vi "Main.vi"(8 "error in (no error)":errorcluster, 11 "Transceiver Thread in":refnum<class "Transceiver Thread.lvclass">) -> (0 "error out":errorcluster, 3 "Transceiver Thread out":refnum<class "Transceiver Thread.lvclass">)   [LabVIEW 2017, in "DSF Core.lvlib" / "Transceiver Thread.lvclass"]
uses:
  Transceiver Thread.lvclass
  C:/Git/DSF/Core/Classes/Thread/Plugin/Plugin Thread.lvclass
  C:/Git/DSF/Core/Classes/Thread/Thread.lvclass
  Thread.lvclass
  Plugin Thread.lvclass
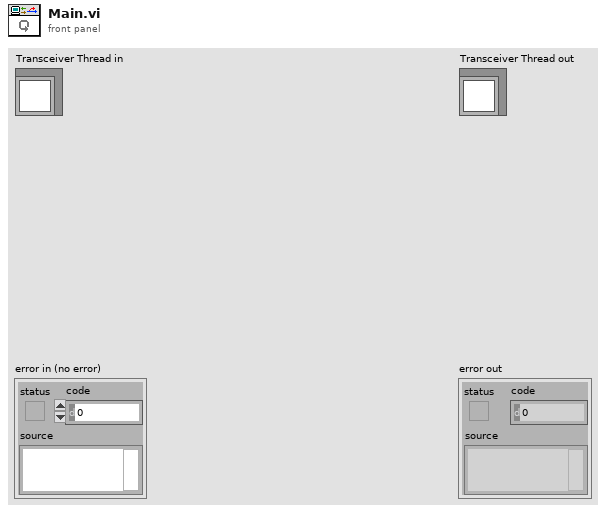
[diagram p1: front panel]
types:
  T1 = typedef "DSF Core.lvlib/Plugin Thread.lvclass/Command Data.ctl" = cluster{"Command":T2, "Parameters":T3}
  T2 = typedef "DSF Core.lvlib/Plugin Thread.lvclass/Commands.ctl" = enum8{"Idle", "Error", "Start", "Rx", "Tx", "Shutdown"}
  T3 = typedef "DSF Core.lvlib/Plugin Interface.lvclass/Command Parameters.ctl" = cluster{"arg1":u64, "arg2":u64}
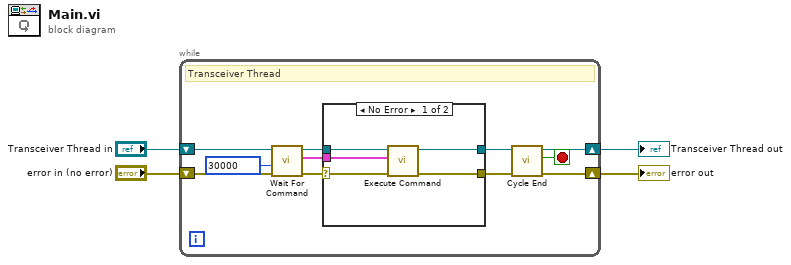
[diagram p0: block diagram]
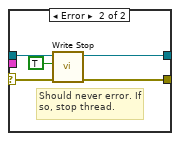
[diagram p2: hidden frame]
diagram:
  n1 = while {
    shift-right: [w8] -> w3
    shift-left: "error in (no error)" -> [w15]
    shift-right: [w10] -> w4
    shift-left: "Transceiver Thread in" -> [w14]
    stop <- w6 stop-if-true
    # "Transceiver Thread"
    n2 = call "Wait For Command.vi"("error in (no error)"=w15, "timeout in ms (0)"=30000 ("timeout in ms"), "Plugin Thread in"=w14) -> ("error out"=w5:errorcluster, "command"=w11:T1, "Plugin Thread out"=w12:refnum<class "Transceiver Thread.lvclass">)  [unwired: 6 in]
    n3 = case shown="No Error" w5 {
      selector: w5 -> [w18 w23]
      tunnel: w12 -> [w19 w24]
      tunnel: [w16 w22] -> w9
      tunnel: w11 -> [w20 _]
      tunnel: [w17 w21] -> w7
      frame No Error {
        n4 = call "Execute Command.vi"("error in (no error)"=w18, "command"=w20, "Transceiver Thread in"=w19) -> ("error out"=w17:errorcluster, "Transceiver Thread out"=w16:refnum<class "Transceiver Thread.lvclass">)  [unwired: 7 in]
      }
      frame Error {
        # "Should never error. If so, stop thread."
        n5 = call "Write Stop.vi"("error in (no error)"=w23, "stop"=TRUE, "Thread in"=w24) -> ("error out"=w21:errorcluster, "Thread out"=w22:refnum<class "Transceiver Thread.lvclass">)  [unwired: 7 in]
      }
    }
    n6 = call "Cycle End.vi"("error in (no error)"=w7, "Plugin Thread in"=w9) -> ("error out"=w8:errorcluster, "stop"=w6:bool, "Plugin Thread out"=w10:refnum<class "Transceiver Thread.lvclass">)  [unwired: 7 in]
  }
  "error out" <- w3
  "Transceiver Thread out" <- w4
